vi "Main.vi"(11 "Script Strategy in":refnum<class "Script Strategy.lvclass">) -> ()   [LabVIEW 2021, in "_Template.lvlib" / "Script Strategy.lvlib" / "Script Strategy.lvclass"]
uses:
  Script Strategy.lvclass
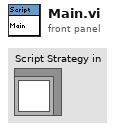
[diagram p1: front panel]
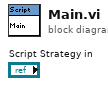
[diagram p0: block diagram]
diagram:
